vi "Configure Voltage.vi"(8 "error in (no error)":errorcluster, 10 "Voltage":dbl, 11 "Agilent 6xxx in":refnum<class "Agilent 6xxx.lvclass">) -> (0 "error out":errorcluster, 3 "Agilent 6xxx out":refnum<class "Agilent 6xxx.lvclass">)   [LabVIEW 2020, in "Agilent 6xxx.lvclass"]
uses:
  Agilent 6xxx.lvclass
  C:/Sandbox/RF Bench/Source Code/WiSpry Test Framework/Instruments/Instrument.lvclass
  C:/Sandbox/RF Bench/Source Code/WiSpry Test Framework/Instruments/Power Supply/Power Supply.lvclass
  Power Supply.lvclass/Power Supply.ctl
  Instrument.lvclass/Instrument.ctl
  Power Supply.lvclass
  Instrument.lvclass
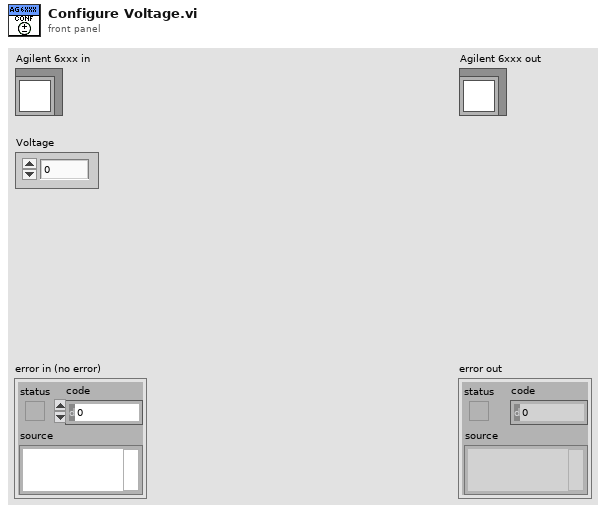
[diagram p1: front panel]
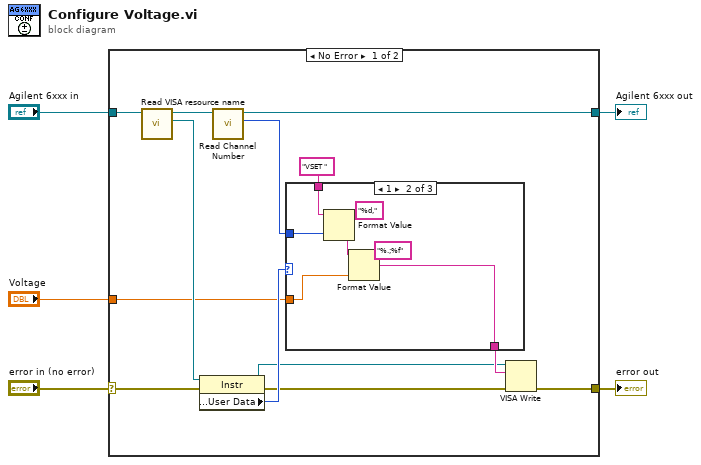
[diagram p0: block diagram]
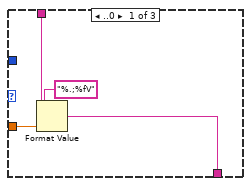
[diagram p2: hidden frame]
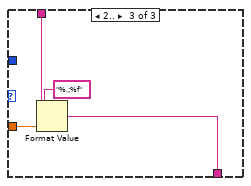
[diagram p3: hidden frame]
diagram:
  n1 = case shown="No Error" "error in (no error)" {
    selector: "error in (no error)" -> [w10 w34]
    tunnel: [w16 w35] -> w4
    tunnel: "Agilent 6xxx in" -> [w17 w35]
    tunnel: [w8 w34] -> w5
    tunnel: "Voltage" -> [w7 _]
    frame No Error {
      n2 = call "Read VISA resource name.vi"("Instrument in"=w17) -> ("VISA resource name"=w9:refnum<visa-resource-name>, "Instrument out"=w18:refnum<class "Agilent 6xxx.lvclass">)  [unwired: 9 in]
      n3 = property class="Instr"(reference=w9, error in=w10) -> (reference out=w12:refnum<visa-resource-name>, error out=w11:errorcluster, "General Settings:User Data"=w13:u32)
      n4 = call "Read Channel Number.vi"("Power Supply in"=w18) -> ("Channel Number"=w6:u8, "Power Supply out"=w16:refnum<class "Agilent 6xxx.lvclass">)  [unwired: 9 in]
      n5 = case shown="1" w13 {
        tunnel: "VSET " -> [w21 w28 w32]
        tunnel: [w20 w23 w31] -> w15
        tunnel: w7 -> [w19 w25 w30]
        tunnel: w6 -> [_ w24 _]
        frame ..0 {
          n6 = Format Value(string ("")=w21, format string="%.;%fV", value (0)=w19) -> (output string=w20:string)
        }
        frame 1 {
          n7 = Format Value(string ("")=w28, format string="%d,", value (0)=w24) -> (output string=w26:string)
          n8 = Format Value(string ("")=w26, format string="%.;%f", value (0)=w25) -> (output string=w23:string)
        }
        frame 2.. {
          n9 = Format Value(string ("")=w32, format string="%.;%f", value (0)=w30) -> (output string=w31:string)
        }
      }
      n10 = VISA Write(VISA resource name=w12, write buffer=w15, error in (no error)=w11) -> (error out=w8:errorcluster)  [unwired: 2 out]
    }
    frame Error {
    }
  }
  "error out" <- w5
  "Agilent 6xxx out" <- w4
